vi "Connect.vi"(8 "error in (no error)":errorcluster, 11 "Videoscan in":refnum<class "Videoscan.lvclass">) -> (0 "error out":errorcluster, 3 "Videoscan out":refnum<class "Videoscan.lvclass">)   [LabVIEW 2014, in "Videoscan.lvclass"]
uses:
  Videoscan.lvclass
  VideoScanLibrary/VideoScanDeviceLibrary.lvclass
  Videoscan.lvclass/Videoscan.ctl
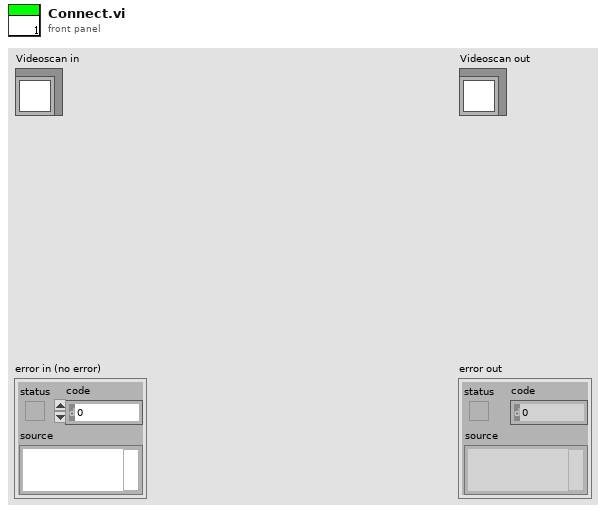
[diagram p1: front panel]
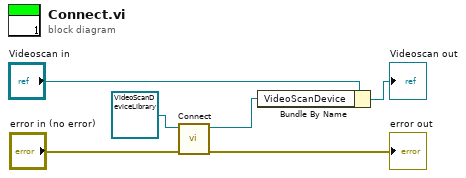
[diagram p0: block diagram]
diagram:
  n1 = call "Connect.vi"("error in (no error)"="error in (no error)", "VideoScanCamera in"=refnum<class "VideoScanDeviceLibrary.lvclass"> refnum ("VideoScanDeviceLibrary.lvclass")) -> ("error out"=→"error out":errorcluster, "VideoScanCamera out"=w2:refnum<class "VideoScanDeviceLibrary.lvclass">)  [unwired: 8 in]
  n2 = Bundle By Name(cluster="Videoscan in", "VideoScanDevice"=w2) -> (→"Videoscan out":refnum<class "Videoscan.lvclass">)
